vi "IDD over Temp.vi"() -> ()   [LabVIEW 2020]
panel:
  in  "Thermostream":refnum<visa-resource-name>="GPIB0::11::INSTR"
  out "error out":errorcluster
  out "IDD":dbl[](array[numeric])
  in  "Multimetru":refnum<visa-resource-name>="GPIB0::24::INSTR"
  in  "SMU":refnum<visa-resource-name>="GPIB0::1::INSTR"
  in  "error in (no error)":errorcluster
  in  "Temperaturi":dbl[](array[numeric])=[-40.0, 25.0, 80.0, 125.0]
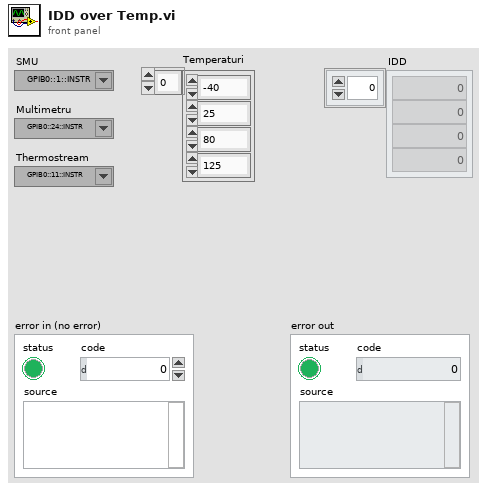
[diagram p1: front panel]
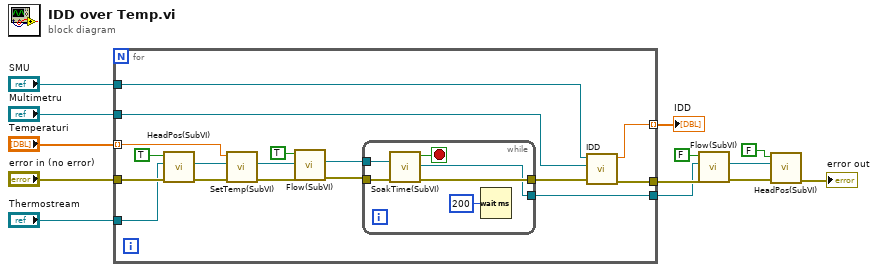
[diagram p0: block diagram]
diagram:
  n1 = for {
    tunnel: "Temperaturi" -> [w27] mode=indexing
    tunnel: "error in (no error)" -> [w30]
    tunnel: "SMU" -> [w22]
    tunnel: "Multimetru" -> [w21]
    tunnel: [w20] -> w8 mode=indexing
    tunnel: [w19] -> w7
    tunnel: "Thermostream" -> [w18]
    tunnel: [w14] -> w2
    n2 = call "HeadPos(SubVI).vi"("error in (no error)"=w30, "VISA resource name"=w18, "Checkbox"=TRUE) -> ("error out"=w28:errorcluster, "VISA resource name 2"=w17:refnum<visa-resource-name>)  [unwired: 7 in]
    n3 = call "SetTemp(SubVI).vi"("error in (no error)"=w28, "VISA resource name"=w17, "Temp"=w27) -> ("error out"=w26:errorcluster, "VISA resource name out"=w16:refnum<visa-resource-name>)  [unwired: 7 in]
    n4 = call "Flow(SubVI).vi"("error in (no error)"=w26, "VISA resource name"=w16, "Checkbox"=TRUE) -> ("error out"=w25:errorcluster, "VISA resource name 2"=w15:refnum<visa-resource-name>)  [unwired: 7 in]
    n5 = while {
      tunnel: [w34] -> w23
      tunnel: w25 -> [w35]
      tunnel: w15 -> [w32]
      tunnel: [w31] -> w14
      stop <- w33 stop-if-true
      n6 = call "SoakTime(SubVI).vi"("error in (no error)"=w35, "VISA resource name"=w32) -> ("error out"=w34:errorcluster, "VISA resource name out"=w31:refnum<visa-resource-name>, "soaked?"=w33:bool)  [unwired: 7 in]
      n7 = Wait (ms)(milliseconds to wait=u32 200) -> ()  [unwired: 1 out]
    }
    n8 = call "IDD.vi"("error in (no error)"=w23, "Multimetru"=w21, "SMU"=w22) -> ("error out"=w19:errorcluster, "IDD"=w20:dbl)  [unwired: 7 in]
  }
  "IDD" <- w8
  n9 = call "Flow(SubVI).vi"("error in (no error)"=w7, "VISA resource name"=w2, "Checkbox"=FALSE) -> ("error out"=w6:errorcluster, "VISA resource name 2"=w1:refnum<visa-resource-name>)  [unwired: 7 in]
  n10 = call "HeadPos(SubVI).vi"("error in (no error)"=w6, "VISA resource name"=w1, "Checkbox"=FALSE) -> ("error out"=→"error out":errorcluster)  [unwired: 7 in, 1 out]
